vi "[Global]VisionAnalysis_DVR.vi"() -> ()   [LabVIEW 2019]
uses:
  VisionAnalysisFramework/PackedLibrary/VisionAnalysisFramework.lvlibp/VisionAnalysisFramework/Object/VisionAnalysisFramework.lvclass
panel:
  in  "VisionAnalysis_DVR":refnum<data-value>
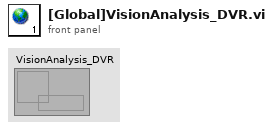
[diagram p1: front panel]
diagram:
